vi "TCP-write.vi"(4 "error in":errorcluster, 5 "Data":string, 6 "Keyword":string, 7 "connection ID":refnum<k5>) -> (0 "error out":errorcluster, 3 "connection ID out":refnum<k5>)   [LabVIEW 2010]
panel:
  in  "timeout ms (10000)":i32=10000
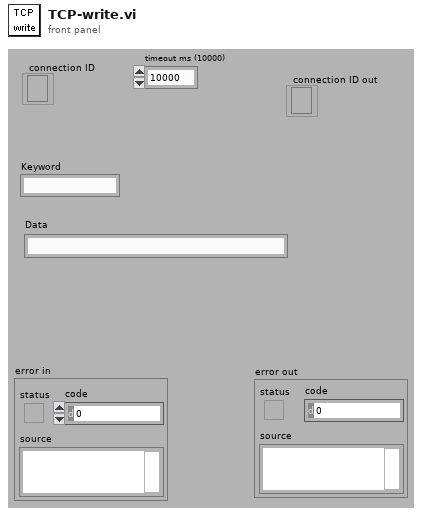
[diagram p1: front panel]
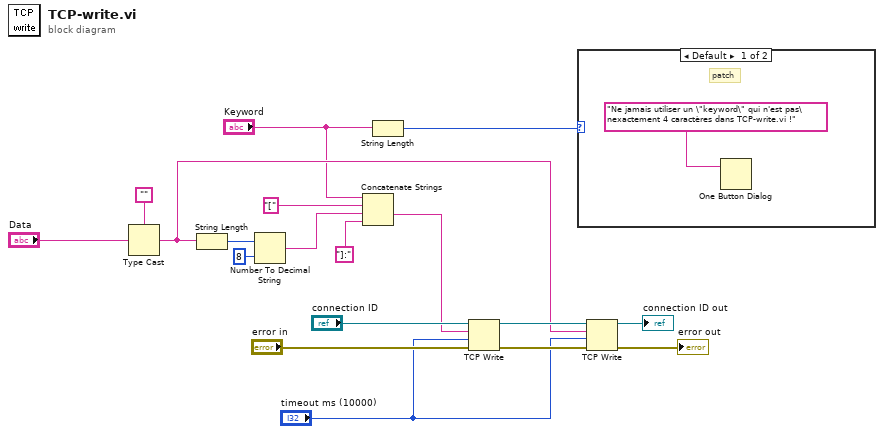
[diagram p0: block diagram]
diagram:
  n1 = Type Cast(type="", x="Data") -> (*(type *) &x=w6:string)
  n2 = String Length(string=w6) -> (length=w13:i32)
  n3 = Number To Decimal String(number=w13, width (-)=i16 8) -> (decimal integer string=w12:string)
  n4 = Concatenate Strings("Keyword", "[", w12, "]:" ("string")) -> (w7:string)
  n5 = String Length(string="Keyword") -> (length=w2:i32)
  n6 = TCP Write(connection ID="connection ID", data in=w7, error in (no error)="error in", 9:"timeout ms (10000)") -> (connection ID out=w9:refnum<k5>, error out=w8:errorcluster)  [unwired: 1 out]
  n7 = case shown="Default" w2 {
    frame Default {
      # "patch"
      n8 = One Button Dialog(message="Ne jamais utiliser un \"keyword\" qui n'est pas\nexactement 4 caractères dans TCP-write.vi !") -> ()  [unwired: 1 in, 1 out]
    }
    frame 4 {
    }
  }
  n9 = TCP Write(connection ID=w9, data in=w6, error in (no error)=w8, 9:"timeout ms (10000)") -> (connection ID out=→"connection ID out":refnum<k5>, error out=→"error out":errorcluster)  [unwired: 1 out]
